vi "Create.vi"(8 "error in (no error)":errorcluster) -> (0 "error out":errorcluster, 3 "Log File Ref":refnum<data-value>)   [LabVIEW 2014, in "Log File.lvclass"]
uses:
  Log File.lvclass
  Log File.lvclass/Log File.ctl
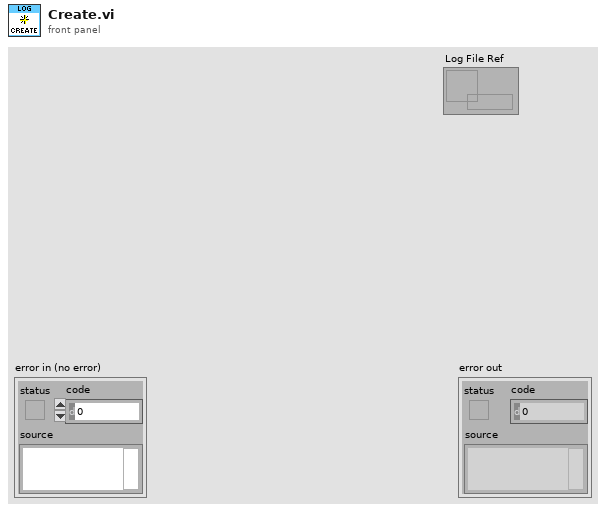
[diagram p1: front panel]
types:
  T1 = enum16{"open", "replace", "create", "open or create", "replace or create", "replace or create with confirmation"}
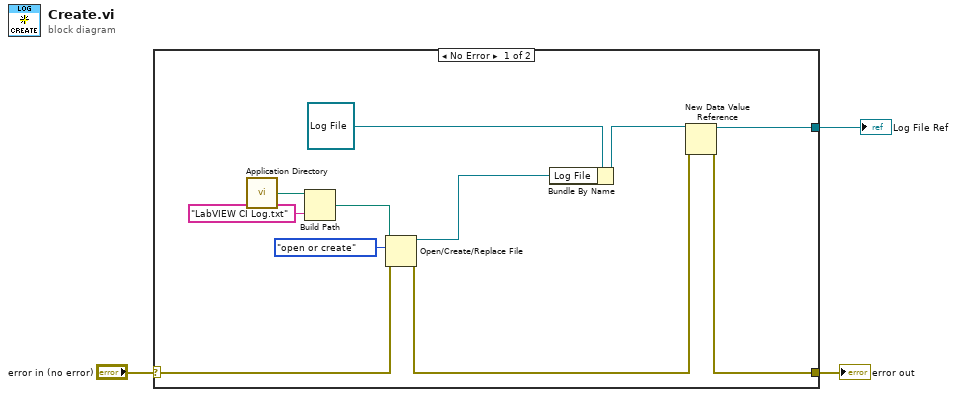
[diagram p0: block diagram]
diagram:
  n1 = case shown="No Error" "error in (no error)" {
    selector: "error in (no error)" -> [w8 w15]
    tunnel: [w13 w15] -> w2
    tunnel: [w14 _] -> w1
    frame No Error {
      n2 = call <vilib>:"Application Directory.vi"() -> ("Application Directory"=w12:path)
      n3 = Build Path(base path=w12, name or relative path="LabVIEW CI Log.txt") -> (appended path=w9:path)
      n4 = Open/Create/Replace File(file path (use dialog)=w9, error in=w8, operation (0:open)=T1."open or create") -> (refnum out=w6:refnum<file>, error out=w7:errorcluster)  [unwired: 3 in, 1 out]
      n5 = Bundle By Name(cluster=refnum<class "Log File.lvclass"> refnum ("Log File in"), "Log File"=w6) -> (w4:refnum<class "Log File.lvclass">)
      n6 = New Data Value Reference(data value=w4, error in=w7) -> (data value reference=w14:refnum<data-value>, error out=w13:errorcluster)
    }
    frame Error {
    }
  }
  "error out" <- w2
  "Log File Ref" <- w1
